vi "Build VIP.vi"(7 "Build number":u32, 8 "error in (no error)":errorcluster, 11 "VIP Path":path) -> (0 "error out":errorcluster)   [LabVIEW 2011]
uses:
  <vilib>/JKI/VIPM API/VIPM API_vipm_api.lvlib
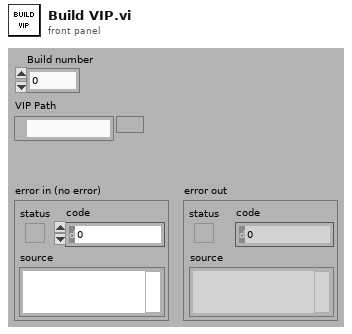
[diagram p1: front panel]
types:
  T1 = typedef "VIPM API_vipm_api.lvlib/VI Package Build Spec Data Cluster_vipm_api.ctl" = cluster{"Package Version":T2, "Product Name":string, "Company Name":string, "Author Name (Person or Company)":string, "Product Homepage (URL)":string, "Legal Copyright":string, "License Agreement Name":string, "Product Description Summary":string, "Product Description":string, "Release Notes - Change Log":string}
  T2 = typedef "VIPM API_vipm_api.lvlib/Version Info Cluster_vipm_api.ctl" = cluster{"major":u32, "minor":u32, "patch":u32, "build":u32}
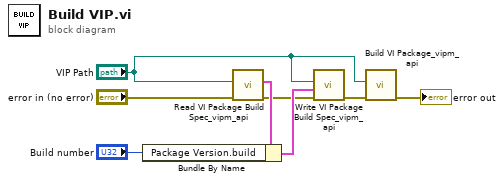
[diagram p0: block diagram]
diagram:
  n1 = call <vilib>:"Read VI Package Build Spec_vipm_api.vi"("error in (no error)"="error in (no error)", "Path to VIPB File"="VIP Path") -> ("error out"=w4:errorcluster, "VI Package Build Spec Data"=w7:T1)  [unwired: 8 in]
  n2 = Bundle By Name(cluster=w7, "Package Version.build"="Build number") -> (w5:T1)
  n3 = call <vilib>:"Write VI Package Build Spec_vipm_api.vi"("error in (no error)"=w4, "VI Package Build Spec Data"=w5, "Path to VIPB File"="VIP Path") -> ("error out"=w3:errorcluster)  [unwired: 8 in]
  n4 = call <vilib>:"Build VI Package_vipm_api.vi"("error in (no error)"=w3, "Path to VIPB File"="VIP Path") -> ("error out"=→"error out":errorcluster)  [unwired: 8 in, 1 out]
